vi "All together.vi"   [LabVIEW 2020]
uses:
  Robot Global Data.vi
types:
  T1 = typedef "WPI_MotorControlDeviceRef.ctl" = cluster{"DeviceStatus":errorcluster, "Type":T2, "PWM":cluster{"PWM Channel":T3, "DeadBand":T4}, "CAN":cluster{"Device Number":u8, "SetOutput VI Ref":variant, "GetOutput VI Ref":variant, "Enable VI Ref":variant, "Disable VI Ref":variant, "Data":variant}, "Invert":bool, "DIO PWM":cluster{"PWM \"Enable\" Channel":T3, "DIOChannel":T5, "PWM Rate":dbl}}
  T2 = typedef "WPI_MotorControlType.ctl" = enum16{"PWM", "CAN", "DIO PWM"}
  T3 = typedef "FPGA_DIOPWMChannel.ctl" = enum8{"PWM 0", "PWM 1", "PWM 2", "PWM 3", "PWM 4", "PWM 5", "PWM 6", "PWM 7", "PWM 8", "PWM 9", "PWM MXP 0", "PWM MXP 1", "PWM MXP 2", "PWM MXP 3", "PWM MXP 4", "PWM MXP 5", "PWM MXP 6", "PWM MXP 7", "PWM MXP 8", "PWM MXP 9", "Invalid"}
  T4 = typedef "WPI_PWMDeadband.ctl" = cluster{"Name":string, "maxPositivePwm":i32, "minPositivePwm":i32, "centerPwm":i32, "maxNegativePwm":i32, "minNegativePwm":i32, "angularRange":u16}
  T5 = typedef "FPGA_DIOChannel.ctl" = enum8{"DIO 0", "DIO 1", "DIO 2", "DIO 3", "DIO 4", "DIO 5", "DIO 6", "DIO 7", "DIO 8", "DIO 9", "DIO MXP 0", "DIO MXP 1", "DIO MXP 2", "DIO MXP 3", "DIO MXP 4", "DIO MXP 5", "DIO MXP 6", "DIO MXP 7", "DIO MXP 8", "DIO MXP 9", "DIO MXP 10", "DIO MXP 11", "DIO MXP 12", "DIO MXP 13", "DIO MXP 14", "DIO MXP 15", "SPI Port CS1", "SPI Port CS2", "SPI Port CS3", "SPI Port MISO", "SPI Port MOSI", "Invalid"}
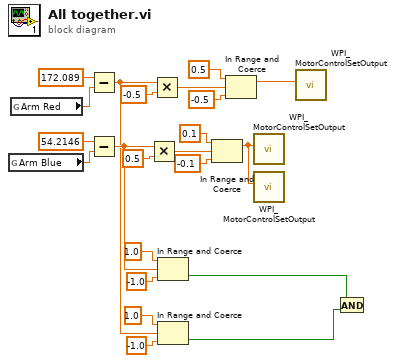
[diagram p0: block diagram]
diagram:
  n1 = global read "Robot Global Data.vi" "Arm Blue"() -> (w9:dbl)
  n2 = global read "Robot Global Data.vi" "Arm Red"() -> (w20:dbl)
  n3 = Subtract(x=172.089, y=w20) -> (x-y=w7:dbl)
  n4 = Subtract(x=54.2146, y=w9) -> (x-y=w8:dbl)
  n5 = Multiply(x=w8, y=0.5) -> (x*y=w17:dbl)
  n6 = Multiply(x=w7, y=-0.5) -> (x*y=w16:dbl)
  n7 = In Range and Coerce(upper limit=1.0, x=w8, lower limit=-1.0) -> (In Range?=w28:bool)  [unwired: 1 out]
  n8 = In Range and Coerce(upper limit=1.0, x=w7, lower limit=-1.0) -> (In Range?=w27:bool)  [unwired: 1 out]
  n9 = In Range and Coerce(upper limit=0.1, x=w17, lower limit=-0.1) -> (coerced(x)=w12:dbl)  [unwired: 1 out]
  n10 = In Range and Coerce(upper limit=0.5, x=w16, lower limit=-0.5) -> (coerced(x)=w13:dbl)  [unwired: 1 out]
  n11 = call <vilib>:"WPI_MotorControlSetOutput.vi"("Output"=w12) -> (3:"MotorControlDevRef"=w1:T1, 11:"MotorControlDevRef"=w5:T1)  [unwired: 7 in, 2 out]
  n12 = call <vilib>:"WPI_MotorControlSetOutput.vi"("Output"=w12) -> (3:"MotorControlDevRef"=w3:T1, 11:"MotorControlDevRef"=w4:T1)  [unwired: 7 in, 2 out]
  n13 = call <vilib>:"WPI_MotorControlSetOutput.vi"("Output"=w13) -> (3:"MotorControlDevRef"=w2:T1, 11:"MotorControlDevRef"=w6:T1)  [unwired: 7 in, 2 out]
  n14 = And(x=w28, y=w27) -> ()  [unwired: 1 out]
